vi "Scatter1010.vi"   [LabVIEW 2013]
uses:
  <vilib>/Heliosphere Research LLC/Advanced Plotting Toolkit/api_plotting/ScatterProperties.ctl
  <vilib>/Heliosphere Research LLC/Advanced Plotting Toolkit/properties/Marker.ctl
  <vilib>/Heliosphere Research LLC/Advanced Plotting Toolkit/properties/Marker_Style.ctl
  <vilib>/Heliosphere Research LLC/Advanced Plotting Toolkit/typedefs/PlotColor.ctl
  <vilib>/Heliosphere Research LLC/Advanced Plotting Toolkit/properties/Line.ctl
  <vilib>/Heliosphere Research LLC/Advanced Plotting Toolkit/properties/Line_Style.ctl
  <vilib>/Heliosphere Research LLC/Advanced Plotting Toolkit/properties/Colormap.ctl
  <vilib>/Heliosphere Research LLC/Advanced Plotting Toolkit/properties/Colormap_Map.ctl
  <vilib>/Heliosphere Research LLC/Advanced Plotting Toolkit/properties/Colormap_Scaling.ctl
  <vilib>/Heliosphere Research LLC/Advanced Plotting Toolkit/properties/Display.ctl
  <vilib>/Heliosphere Research LLC/Advanced Plotting Toolkit/Advanced Plotting Toolkit.lvlib
types:
  T1 = typedef "Advanced Plotting Toolkit.lvlib/Colormap_Map.ctl" = enum16{"Automatic", "Rainbow", "Hot and Cold", "White-Black", "White-Blue", "White-Green", "White-Red", "Fire", "Water", "Earth", "Air", "Pastel", "Banded", "Stepped"}
  T2 = typedef "Advanced Plotting Toolkit.lvlib/ScatterProperties.ctl" = cluster{"Marker":T3, "Line":T6, "Colormap":T8, "Display":T10}
  T3 = typedef "Advanced Plotting Toolkit.lvlib/Marker.ctl" = cluster{"Style":T4, "Color":T5, "Size":dbl}
  T4 = typedef "Advanced Plotting Toolkit.lvlib/Marker_Style.ctl" = enum16{"Automatic", "Circle", "Square", "Triangle", "Diamond", "Star", "Invisible"}
  T5 = typedef "Advanced Plotting Toolkit.lvlib/PlotColor.ctl" = u32
  T6 = typedef "Advanced Plotting Toolkit.lvlib/Line.ctl" = cluster{"Style":T7, "Color":T5, "Width":sgl}
  T7 = typedef "Advanced Plotting Toolkit.lvlib/Line_Style.ctl" = enum16{"Automatic", "Solid", "Dashed", "Dotted", "Dash-dot", "Invisible"}
  T8 = typedef "Advanced Plotting Toolkit.lvlib/Colormap.ctl" = cluster{"Map":T1, "Value Min":dbl, "Value Max":dbl, "Scaling":T9, "Reverse":bool}
  T9 = typedef "Advanced Plotting Toolkit.lvlib/Colormap_Scaling.ctl" = enum16{"Default"}
  T10 = typedef "Advanced Plotting Toolkit.lvlib/Display.ctl" = cluster{"Alpha":dbl, "Z Order":dbl}
  T11 = typedef "Advanced Plotting Toolkit.lvlib/PlotID.ctl" = i32
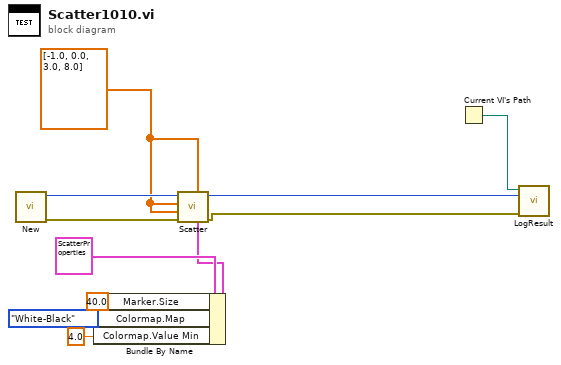
[diagram p0: block diagram]
diagram:
  w3 = dbl[] [-1.0, 0.0, 3.0, 8.0] ("X Data")
  n1 = call <vilib>:"New.vi"() -> ("error out"=w9:errorcluster, "Plot ID"=w10:T11)  [unwired: 10 in]
  n2 = Bundle By Name(cluster=T2 {"Marker"={"Style"=enum."Automatic", "Color"=2147483647, "Size"=nan}, "Line"={"Style"=enum."Automatic", "Color"=2147483647, "Width"=nan}, "Colormap"={"Map"=enum."Automatic", "Value Min"=nan, "Value Max"=nan, "Scaling"=enum."Default", "Reverse"=FALSE}, "Display"={"Alpha"=nan, "Z Order"=nan}} ("Scatter Properties"), "Marker.Size"=40.0, "Colormap.Map"=Colormap_Map."White-Black", "Colormap.Value Min"=4.0) -> (w5:T2)
  n3 = call <vilib>:"Scatter.vi"("Properties"=w5, "Colormap Values"=w3, "error in (no error)"=w9, "Y Data"=w3, "X Data"=w3, "Plot ID"=w10) -> ("error out"=w7:errorcluster, "Plot ID Out"=w8:T11)  [unwired: 4 in]
  n4 = Current VI's Path() -> (path=w11:path)
  n5 = call "LogResult.vi"("Test Result"=w7, "Test Artifact"=w8, "VI Path"=w11) -> ()  [unwired: 9 in]
